vi "load2table.vi"(1 "Table":refnum<vi>, 2 "Array":string[][](array[string])) -> (0 "Rows":i32)   [LabVIEW 2010]
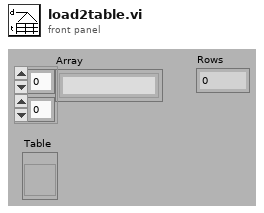
[diagram p1: front panel]
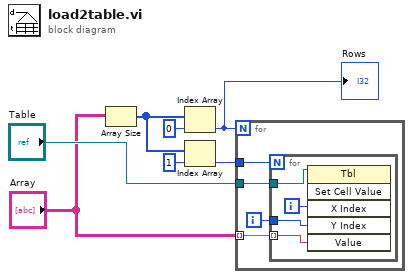
[diagram p0: block diagram]
diagram:
  n1 = Array Size(array="Array") -> (size(s)=w5:i32[])
  n2 = Index Array(array=w5, index=0) -> (element=w1:i32)
  "Rows" <- w1
  n3 = Index Array(array=w5, index=1) -> (element=w6:i32)
  n4 = for {
    N: w1 -> [_]
    tunnel: "Array" -> [w10] mode=indexing
    tunnel: w6 -> [w11]
    tunnel: "Table" -> [w8]
    i -> [w9]
    n5 = for {
      N: w11 -> [_]
      tunnel: w10 -> [w15] mode=indexing
      tunnel: w9 -> [w13]
      tunnel: w8 -> [w12]
      i -> [w14]
      n6 = invoke on="Invoke Node" class="Tbl" method="Set Cell Value"(reference=w12, "X Index"=w14, "Y Index"=w13, "Value"=w15) -> ()  [unwired: 2 in, 6 out]
    }
  }
